vi "main.vi"() -> ()   [LabVIEW 2024]
panel:
  in  "stop":bool
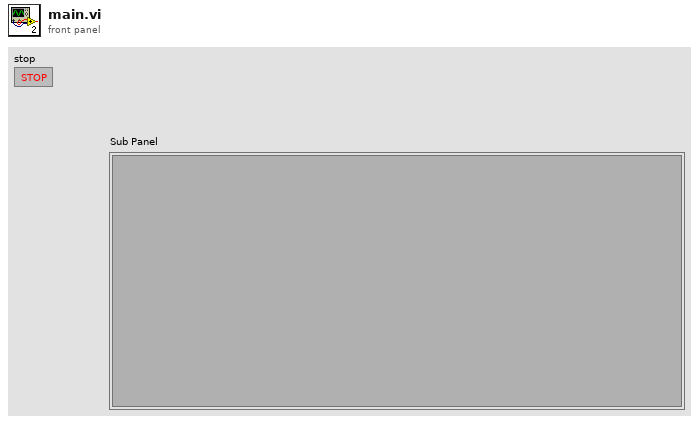
[diagram p1: front panel]
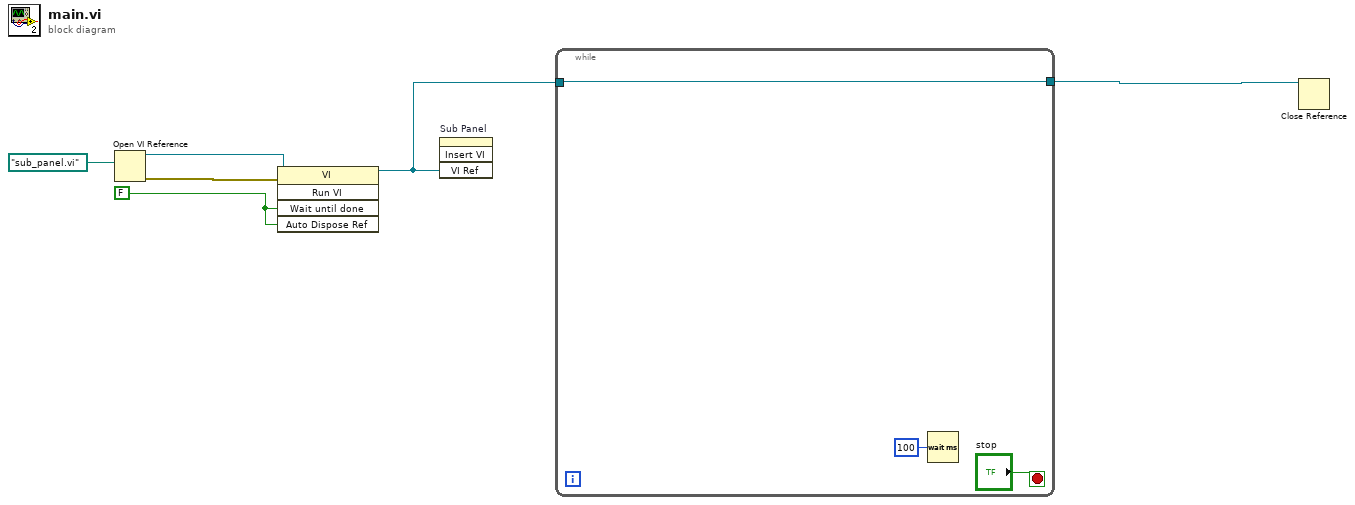
[diagram p0: block diagram]
diagram:
  w3 = FALSE ("Wait Until Done")
  n1 = Open VI Reference(vi path=path "sub_panel.vi") -> (vi reference=w5:refnum<vi>, error out=w4:errorcluster)  [unwired: 5 in]
  n2 = invoke class="VI" method="Run VI"(reference=w5, error in=w4, "Wait until done"=w3, "Auto Dispose Ref"=w3) -> (reference out=w2:refnum<vi>)  [unwired: 1 in, 4 out]
  n3 = invoke on="Sub Panel" class="SubPnl" method="Insert VI"("VI Ref"=w2) -> ()  [unwired: 3 in, 4 out]
  n4 = while {
    tunnel: w2 -> [w8]
    tunnel: [w8] -> w1
    stop <- "stop" stop-if-true
    n5 = Wait (ms)(milliseconds to wait=u32 100) -> ()  [unwired: 1 out]
  }
  n6 = Close Reference(reference=w1) -> ()  [unwired: 1 in, 1 out]
